vi "OpenConnection.vi"(8 "error in (no error)":errorcluster, 9 "remote port or service name":u16=10001, 10 "address":string="192.168.1.11", 11 "TCP Connection in":refnum<class "TCP Connection.lvclass">) -> (0 "error out":errorcluster, 3 "TCP Connection out":refnum<class "TCP Connection.lvclass">)   [LabVIEW 2011, in "TCP Connection.lvclass"]
uses:
  TCP Connection.lvclass
  TCP Connection.lvclass/TCP Connection.ctl
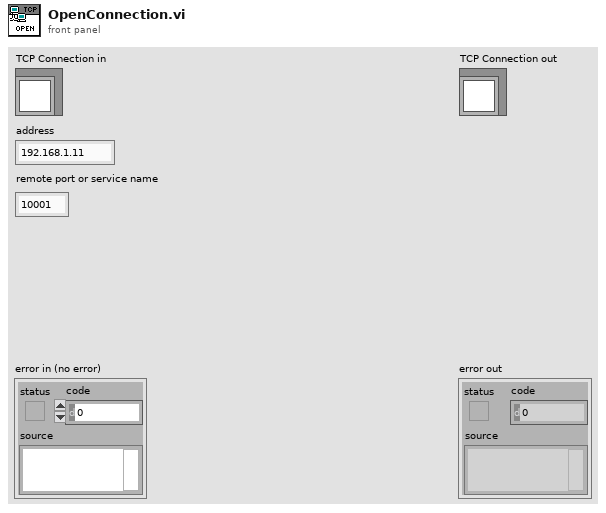
[diagram p1: front panel]
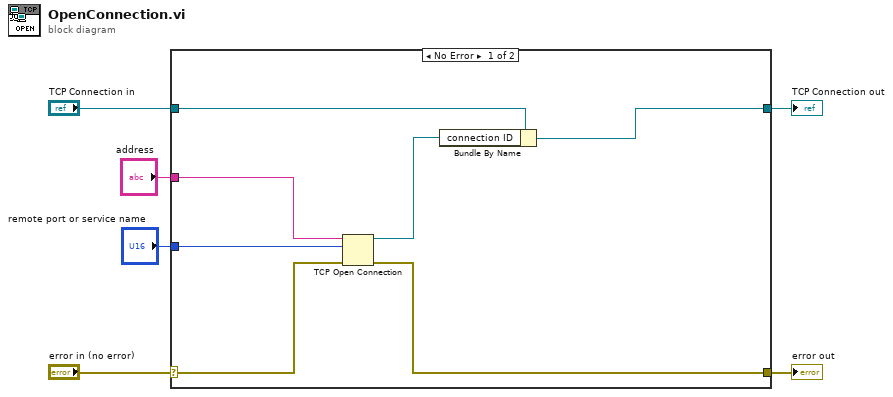
[diagram p0: block diagram]
diagram:
  n1 = case shown="No Error" "error in (no error)" {
    selector: "error in (no error)" -> [w13 w15]
    tunnel: [w7 w15] -> w5
    tunnel: [w8 w14] -> w3
    tunnel: "TCP Connection in" -> [w10 w14]
    tunnel: "remote port or service name" -> [w12 _]
    tunnel: "address" -> [w11 _]
    frame No Error {
      n2 = TCP Open Connection(address=w11, remote port or service name=w12, error in (no error)=w13) -> (connection ID=w9:refnum<k5>, error out=w7:errorcluster)  [unwired: 2 in]
      n3 = Bundle By Name(cluster=w10, "connection ID"=w9) -> (w8:refnum<class "TCP Connection.lvclass">)
    }
    frame Error {
    }
  }
  "error out" <- w5
  "TCP Connection out" <- w3
